vi "setUp.vi"(8 "error in (no error)":errorcluster, 11 "reference in":refnum<class "Test TCP Caller Endpoint Disconnect.lvclass">) -> (0 "error out":errorcluster, 3 "reference out":refnum<class "Test TCP Caller Endpoint Disconnect.lvclass">)   [LabVIEW 2020, in "Test TCP Caller Endpoint Disconnect.lvclass"]
doc: "setUp runs prior to the test method during test execution. Use this method to initialize any object data required by your tests."
uses:
  Test TCP Caller Endpoint Disconnect.lvclass
  <vilib>/addons/_JKI Toolkits/VI Tester/TestCase.llb/TestCase.lvclass
  <vilib>/ActorFramework/Actor/Actor.lvclass
  <vilib>/ActorFramework/Message Queue/Message Queue.lvclass
  Source/Protocols/TCP Strategy/TCP Stream Listener/TCP Stream Listener.lvclass
  Source/Protocols/TCP Strategy/TCP Stream Initiator/TCP Stream Initiator.lvclass
  Source/Protocols/TCP Strategy/TCP Stream/TCP Stream.lvclass
  Source/Ciphers/AES/AES.lvclass
  Source/Ciphers/AES/Ton Plomp Encryption/AES-Modes.ctl
  Source/Ciphers/AES/Ton Plomp Encryption/Encryption.lvlib
  Source/Nested Endpoint/Nested Endpoint/Nested Endpoint.lvclass
  Source/Network Endpoint/Network Endpoint/Network Endpoint.lvclass
  Source/Caller Endpoint/Caller Endpoint/Caller Endpoint.lvclass
  Support/Caller Test Harness/Caller Test Harness/Caller Test Harness.lvclass
  Source/Abstract Classes/Message Stream/Message Stream.lvclass
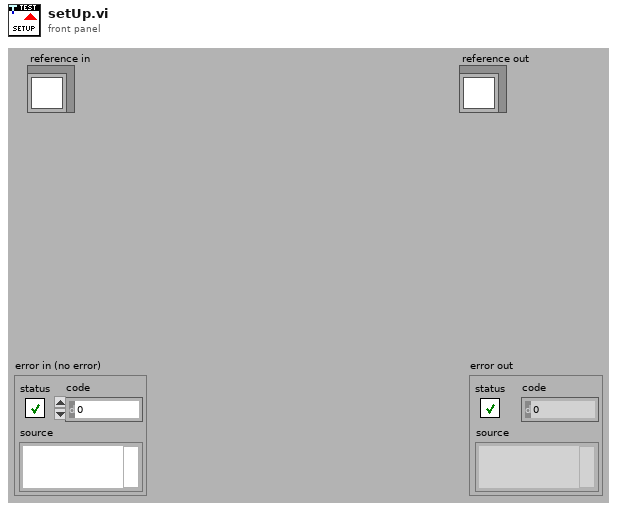
[diagram p1: front panel]
types:
  T1 = typedef "Encryption.lvlib/AES-Modes.ctl" = enum16{"ECB", "CBC", "CFB128", "OFB"}
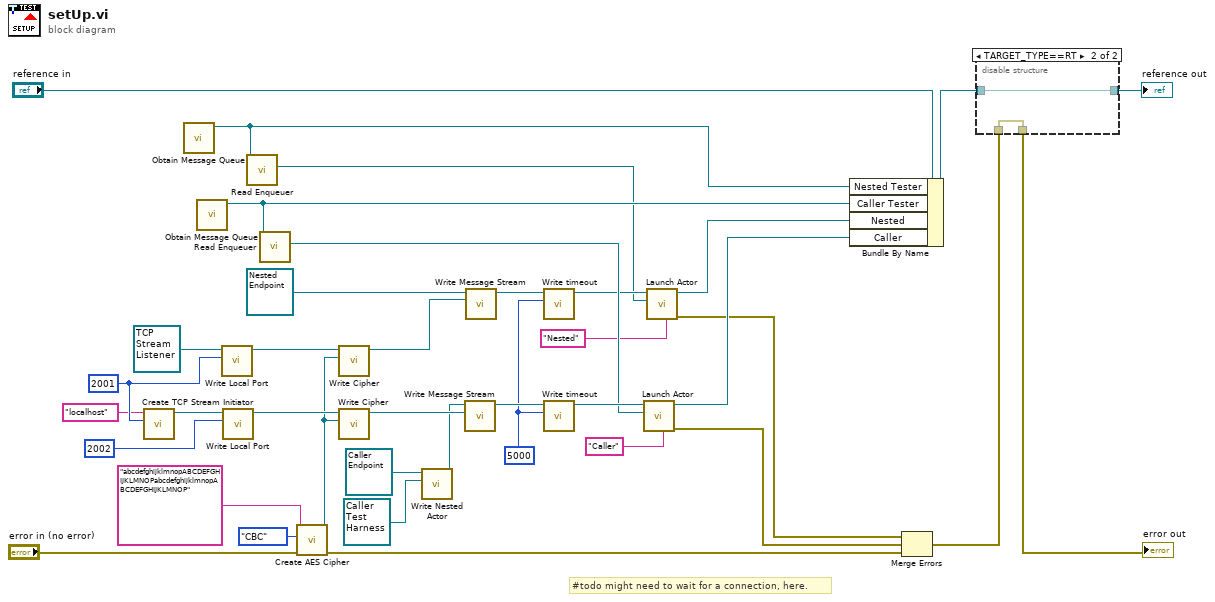
[diagram p0: block diagram]
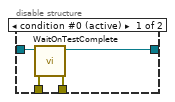
[diagram p2: hidden frame]
diagram:
  w16 = 5000 ("timeout")
  w32 = u16 2001 ("Port")
  # "#todo might need to wait for a connection, here."
  n1 = call "Create TCP Stream Initiator.vi"("Remote Port"=w32, "Remote Address"="localhost" ("IP Address")) -> ("TCP Stream Initiator"=w34:refnum<class "TCP Stream Initiator.lvclass">)  [unwired: 9 in]
  n2 = call <vilib>:"Obtain Message Queue.vi"() -> ("Message Queue"=w2:refnum<class "Message Queue.lvclass">)  [unwired: 10 in, 1 out]
  n3 = call <vilib>:"Obtain Message Queue.vi"() -> ("Message Queue"=w20:refnum<class "Message Queue.lvclass">)  [unwired: 10 in, 1 out]
  n4 = call "Write Local Port.vi"("local port"=w32, "TCP Stream in"=refnum<class "TCP Stream Listener.lvclass"> refnum ("TCP Stream Listener.lvclass")) -> ("TCP Stream out"=w31:refnum<class "TCP Stream Listener.lvclass">)  [unwired: 9 in]
  n5 = call "Write Local Port.vi"("local port"=u16 2002, "TCP Stream in"=w34) -> ("TCP Stream out"=w30:refnum<class "TCP Stream Initiator.lvclass">)  [unwired: 9 in]
  n6 = call <vilib>:"Read Enqueuer.vi"("Message Queue"=w2) -> ("Message Enqueuer"=w1:refnum<class "Message Enqueuer.lvclass">)  [unwired: 10 in]
  n7 = call <vilib>:"Read Enqueuer.vi"("Message Queue"=w20) -> ("Message Enqueuer"=w9:refnum<class "Message Enqueuer.lvclass">)  [unwired: 10 in]
  n8 = call "Create AES Cipher.vi"("error in (no error)"="error in (no error)", "Operation Mode"=AES-Modes."CBC", "Cipher Key"="abcdefghijklmnopABCDEFGHIJKLMNOPabcdefghijklmnopABCDEFGHIJKLMNOP") -> ("error out"=w26:errorcluster, "AES out"=w25:refnum<class "AES.lvclass">)  [unwired: 7 in]
  n9 = call "Write Cipher.vi"("Cipher"=w25, "Message Stream in"=w31) -> ("Message Stream out"=w23:refnum<class "TCP Stream Listener.lvclass">)  [unwired: 9 in]
  n10 = call "Write Cipher.vi"("Cipher"=w25, "Message Stream in"=w30) -> ("Message Stream out"=w22:refnum<class "TCP Stream Initiator.lvclass">)  [unwired: 9 in]
  n11 = call "Write Nested Actor.vi"("Nested Actor"=refnum<class "Caller Test Harness.lvclass"> refnum ("Caller Test Harness.lvlib:Caller Test Harness.lvclass"), "Caller Endpoint in"=refnum<class "Caller Endpoint.lvclass"> refnum ("Caller Endpoint.lvlib:Caller Endpoint.lvclass")) -> ("Caller Endpoint out"=w14:refnum<class "Caller Endpoint.lvclass">)  [unwired: 9 in]
  n12 = call "Write Message Stream.vi"("Message Stream"=w22, "Network Endpoint in"=w14) -> ("Network Endpoint out"=w17:refnum<class "Caller Endpoint.lvclass">)  [unwired: 9 in]
  n13 = call "Write Message Stream.vi"("Message Stream"=w23, "Network Endpoint in"=refnum<class "Nested Endpoint.lvclass"> refnum ("Nested Endpoint.lvlib:Nested Endpoint.lvclass")) -> ("Network Endpoint out"=w18:refnum<class "Nested Endpoint.lvclass">)  [unwired: 9 in]
  n14 = call "Write timeout.vi"("timeout"=w16, "Network Endpoint in"=w18) -> ("Network Endpoint out"=w6:refnum<class "Nested Endpoint.lvclass">)  [unwired: 9 in]
  n15 = call "Write timeout.vi"("timeout"=w16, "Network Endpoint in"=w17) -> ("Network Endpoint out"=w12:refnum<class "Caller Endpoint.lvclass">)  [unwired: 9 in]
  n16 = call <vilib>:"Launch Actor.vi"("Debug Alias"="Caller", "Actor-to-Caller Enqueuer"=w9, "Actor"=w12) -> ("error out"=w7:errorcluster, "Caller-To-Actor Enqueuer"=w11:refnum<class "Message Enqueuer.lvclass">)  [unwired: 7 in]
  n17 = call <vilib>:"Launch Actor.vi"("Debug Alias"="Nested", "Actor-to-Caller Enqueuer"=w1, "Actor"=w6) -> ("error out"=w3:errorcluster, "Caller-To-Actor Enqueuer"=w5:refnum<class "Message Enqueuer.lvclass">)  [unwired: 7 in]
  n18 = Bundle By Name(cluster="reference in", "Nested Tester"=w2, "Caller Tester"=w20, "Nested"=w5, "Caller"=w11) -> (w35:refnum<class "Test TCP Caller Endpoint Disconnect.lvclass">)
  n19 = Merge Errors(w3, w7, w26) -> (w8:errorcluster)
  n20 = disable-structure shown="TARGET_TYPE==RT" {
    disable-tunnel: w8 -> [w42 w43]
    disable-tunnel: [w41 w43] -> w38
    disable-tunnel: [w40 w44] -> w36
    disable-tunnel: w35 -> [w39 w44]
    frame condition #0 (active) {
      n21 = call <vilib>:"WaitOnTestComplete.vi"("error in (no error)"=w42, "TestCase in"=w39) -> ("error out"=w41:errorcluster, "TestCase out"=w40:refnum<class "Test TCP Caller Endpoint Disconnect.lvclass">)  [unwired: 8 in]
    }
    frame condition #1 {
    }
  }
  "error out" <- w38
  "reference out" <- w36
